vi "VisionTargetDataType.vi"(6 "height":dbl, 8 "orientation":dbl, 9 "y":dbl, 10 "x":dbl, 11 "Name":string) -> (2 "Target":T1)   [LabVIEW 2018]
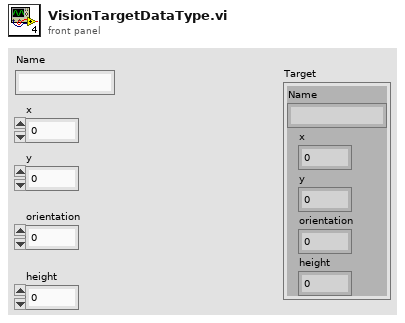
[diagram p1: front panel]
types:
  T1 = cluster{"Name":string, "x":dbl, "y":dbl, "orientation":dbl, "height":dbl}
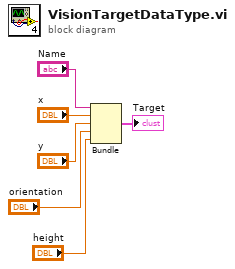
[diagram p0: block diagram]
diagram:
  n1 = Bundle("Name"="Name", "x"="x", "y"="y", "orientation"="orientation", "height"="height") -> (→"Target":T1)  [unwired: 1 in]
